vi "Scanner-XYZMove.vi"(5 "加速度":dbl=900.0, 7 "最高速":dbl=1000.0, 8 "Error In":errorcluster, 11 "X-Y-Z移動":dbl[](array[numeric])=[0.0, 0.0, 0.0]) -> (0 "Error Out":errorcluster, 1 "辨識結果(包含位置)":cluster{"讀取到時的位子":dbl, "辨識結果":string}[](array[cluster]), 2 "讀取到時的位子":dbl[](array[numeric]), 3 "辨識結果":string[](array[string]), 4 "辨識數量":i32, 6 "讀取機率":i32[](array[numeric]))   [LabVIEW 2019]
uses:
  <vilib>/Platform/TimedLoop/XDataNode/timing_clust.ctl
  <vilib>/Platform/TimedLoop/XDataNode/nitl_modes.ctl
  <vilib>/Platform/TimedLoop/XDataNode/wakeup.ctl
  9317ad16-1364-411d-9d7d-80c797a5b455.vi
  d1461482-5f26-4b15-89db-d86a902074c8.vi
  Variable/Lock-PID.vi
  Variable/Position.vi
  <vilib>/platform/TimedLoop/XDataNode/XDataNode.xnode
  <vilib>/Platform/TimedLoop/XDataNode/XDNodeRunTimeDep.lvlib
panel:
  out "讀取機率(折線圖)":i32[](graph)
  out "讀取機率":dbl[](array[slide]) scale=0.0..10.0
  out "三角形?":bool
  in  "Stop":bool
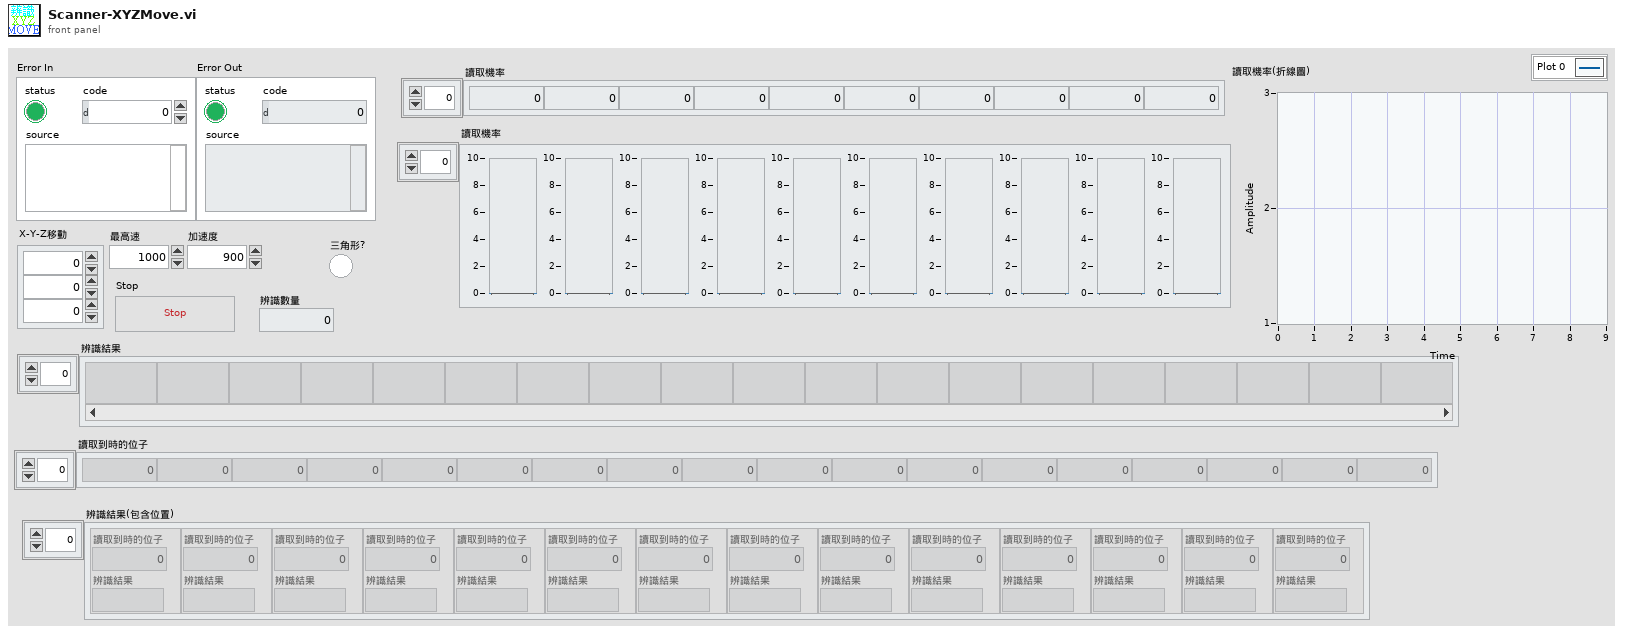
[diagram p1: front panel]
types:
  T1 = typedef "XDNodeRunTimeDep.lvlib/timing_clust.ctl" = cluster{"Expected End [f-1]":u64, "Actual End [f-1]":u64, "Finished Late? [f-1]":bool, "Expected End [i-1]":u64, "Actual End [i-1]":u64, "Finished Late? [i-1]":bool, "Expected Start [i]":u64, "Actual Start [i]":u64, "Expected Start [f]":u64, "Actual Start [f]":u64, "Source Name":string, "Structure Name":string, "Period":i64, "Deadline":i64, "Offset":i64, "Start":i64, "Priority":i32, "Timeout":i32, "Mode":T2, "Wakeup Reason":T3, "Error":errorcluster, "Source Type":string, "Secondary Source Type":string, "Global End Time":u64, "Global Start Time":u64, "Frame Duration":u64, "Iteration Duration":u64, "Assigned CPU":i32, "I/O Scan Engine Mode":u32}
  T2 = typedef "XDNodeRunTimeDep.lvlib/nitl_modes.ctl" = enum32{"No Change", "Process missed periods, maintain original phase", "Discard missed periods, maintain original phase", "Process missed periods, ignore original phase", "Discard missed periods, ignore original phase"}
  T3 = typedef "XDNodeRunTimeDep.lvlib/wakeup.ctl" = enum32{"Normal", "Aborted", "Asynchronous wakeup", "Timing source error", "Timed loop error", "Timeout"}
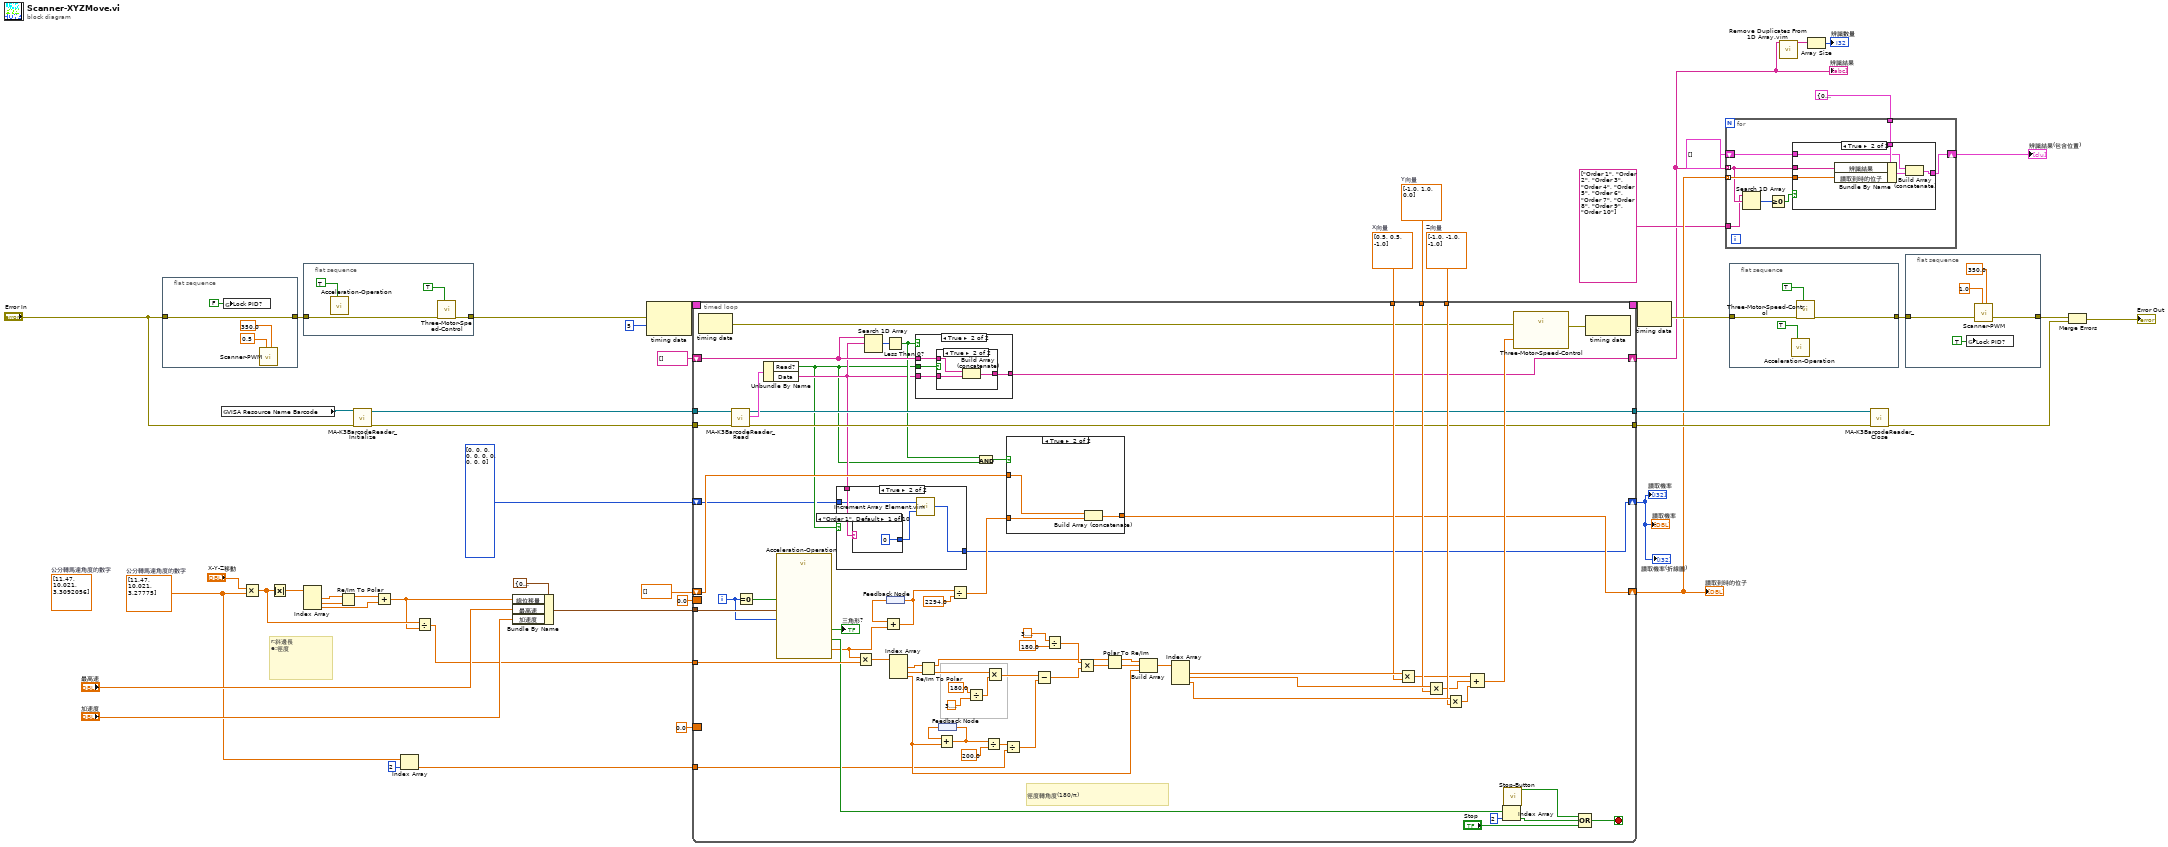
[diagram p0: block diagram]
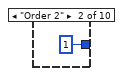
[diagram p4: hidden frame]
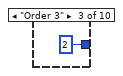
[diagram p5: hidden frame]
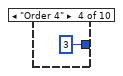
[diagram p6: hidden frame]
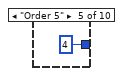
[diagram p7: hidden frame]
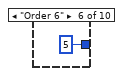
[diagram p8: hidden frame]
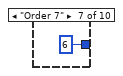
[diagram p9: hidden frame]
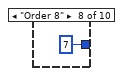
[diagram p10: hidden frame]
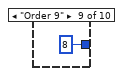
[diagram p11: hidden frame]
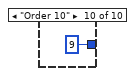
[diagram p12: hidden frame]
diagram:
  (unwired) dbl[] [11.47, 10.021, 3.3092056]  # 公分轉馬達角度的數字
  w29 = dbl[] [-1.0, -1.0, -1.0]  # Z向量
  w30 = dbl[] [-1.0, 1.0, 0.0]  # Y向量
  w31 = dbl[] [0.5, 0.5, -1.0]  # X向量
  w28 = dbl[] [11.47, 10.021, 3.27775]  # 公分轉馬達角度的數字
  # "r:斜邊長\ne:徑度"
  n1 = flat-sequence {
    tunnel: [w52] -> w24
    tunnel: "Error In" -> [w52]
    frame #0 {
      n2 = global write "Lock-PID.vi" "Lock PID?"(FALSE ("Lock PID?")) -> ()
      n3 = call "Scanner-PWM.vi"("Frequency [Hz]"=350.0, "Duty Cycle"=0.5) -> ()  [unwired: 9 in, 1 out]
    }
  }
  n4 = global read "Position.vi" "VISA Resource Name Barcode"() -> (w7:refnum<visa-resource-name>)
  n5 = Multiply(x="X-Y-Z移動", y=w28) -> (x*y=w35:dbl[])
  n6 = Absolute Value(x=w35) -> (abs(x)=w46:dbl[])
  n7 = Index Array(array=w46) -> (element #1=w42:dbl, element #2=w47:dbl, element #3=w43:dbl)  [unwired: 3 in]
  n8 = flat-sequence {
    tunnel: w24 -> [w56]
    tunnel: [w55] -> w34
    frame #0 {
      n9 = call "Acceleration-Operation.vi"("Reset"=TRUE) -> ()  [unwired: 8 in, 3 out]
      n10 = call "Three-Motor-Speed-Control.vi"("Reset"=TRUE, "Error In"=w56) -> ("Error Out"=w55:errorcluster)  [unwired: 9 in]
    }
  }
  n11 = Re/Im To Polar(2:w47, 3:w42) -> (1:w44:dbl)  [unwired: 1 out]
  n12 = call "MA-K3BarcodeReader_Initialize.vi"("Error In"="Error In", "掃碼機串口"=w7) -> ("Error Out"=w15:errorcluster, "VISA Resource"=w14:refnum<visa-resource-name>)  [unwired: 8 in]
  n13 = Add(x=w44, y=w43) -> (x+y=w23:dbl)
  n14 = Index Array(array=w28, index=2) -> (element=w27:dbl)
  n15 = Divide(x=w35, y=w23) -> (x/y=w36:dbl[])
  n16 = Bundle By Name(cluster=cluster{"總位移量":dbl, "最高速":dbl, "加速度":dbl} {"總位移量"=0.0, "最高速"=0.0, "加速度"=0.0} ("計算設置"), "總位移量"=w23, "最高速"="最高速", "加速度"="加速度") -> (w37:cluster{"總位移量":dbl, "最高速":dbl, "加速度":dbl})
  n17 = node-c288(w34, i64 5 ("Period")) -> (w49:T1)
  n18 = timed-loop "Timed Loop" {
    timing: w49 -> [_]
    timing-out: [_] -> w48
    tunnel: w37 -> [w125]
    tunnel: w36 -> [w124]
    border: 0.0 -> [_]
    tunnel: w31 -> [w94]
    tunnel: w30 -> [w92]
    tunnel: w29 -> [w90]
    tunnel: w27 -> [w82]
    border: 0.0 -> [_]
    shift-right: [w73] -> w12
    shift-left: dbl[] [] -> [w72]
    tunnel: [w69] -> w18
    tunnel: [w68] -> w17
    shift-right: [w70] -> w5
    shift-left: string[] [] -> [w65]
    tunnel: w15 -> [w67]
    tunnel: w14 -> [w66]
    shift-right: [w58] -> w1
    shift-left: i32[] [0, 0, 0, 0, 0, 0, 0, 0, 0, 0] -> [w59]
    i -> [w122]
    stop <- w120 stop-if-true
    # "徑度轉角度(180/π)"
    n19 = node-c288() -> (w85:errorcluster)  [unwired: 1 in]
    n20 = call "MA-K3BarcodeReader_Read.vi"("error in (no error)"=w67, "VISA Reference"=w66) -> ("error out"=w69:errorcluster, "Result"=w71:cluster{"Read?":bool, "Data":string}, "VISA Reference"=w68:refnum<visa-resource-name>)  [unwired: 7 in]
    n21 = Equal To 0?(x=w122) -> (x = 0?=w123:bool)
    n22 = Unbundle By Name(w71) -> ("Read?"=w60:bool, "Data"=w61:string)
    n23 = call "Acceleration-Operation.vi"("Reset"=w123, "迴圈( I )"=w122, "計算設置"=w125) -> ("完成?"=w119:bool[], "速度"=w78:dbl, "三角形?"=→"三角形?":bool)  [unwired: 6 in]
    n24 = case shown="True" w60 {
      tunnel: w61 -> [_ w130]
      tunnel: w59 -> [w126 w129]
      tunnel: [w126 w127] -> w58
      frame False {
      }
      frame True {
        n25 = case shown="\"Order 1\", Default" w130 {
          tunnel: [0 1 2 3 4 5 6 7 8 9] -> w128
          frame "Order 1", Default {
          }
          frame "Order 2" {
          }
          frame "Order 3" {
          }
          frame "Order 4" {
          }
          frame "Order 5" {
          }
          frame "Order 6" {
          }
          frame "Order 7" {
          }
          frame "Order 8" {
          }
          frame "Order 9" {
          }
          frame "Order 10" {
          }
        }
        n26 = call "Increment Array Element.vim"("index"=w128, "array in"=w129) -> ("array out"=w127:i32[])
      }
    }
    n27 = Multiply(x=w78, y=w124) -> (x*y=w116:dbl[])
    n28 = Search 1D Array(1D array=w65, element=w61) -> (index of element=w64:i32)  [unwired: 1 in]
    n29 = Less Than 0?(x=w64) -> (x < 0?=w62:bool)
    n30 = feedback #1() -> (w77:dbl)
    n31 = Add(x=w77, y=w78) -> (x+y=w76:dbl)
    n32 = feedback-in #1(w76) -> ()
    n33 = Index Array(array=w116) -> (element #1=w115:dbl, element #2=w114:dbl, element #3=w97:dbl)  [unwired: 3 in]
    n34 = case shown="True" w62 {
      tunnel: w61 -> [_ w145]
      tunnel: w60 -> [_ w144]
      tunnel: [w141 w143] -> w70
      tunnel: w65 -> [w141 w142]
      frame False {
      }
      frame True {
        n35 = case shown="True" w144 {
          tunnel: w145 -> [_ w149]
          tunnel: [w146 w148] -> w143
          tunnel: w142 -> [w146 w147]
          frame False {
          }
          frame True {
            n36 = Build Array (concatenate)(w147, w149) -> (w148:string[])
          }
        }
      }
    }
    n37 = Re/Im To Polar(2:w114, 3:w115) -> (0:w113:dbl, 1:w100:dbl)
    n38 = feedback #2() -> (w109:dbl)
    n39 = Add(x=w109, y=w97) -> (x+y=w108:dbl)
    n40 = feedback-in #2(w108) -> ()
    n41 = Divide(x=w76, y=2294.0) -> (x/y=w74:dbl)
    n42 = Divide(x=180.0, y=3.141592653589793) -> (x/y=w110:dbl)
    n43 = And(x=w62, y=w60) -> (x .and. y?=w63:bool)
    n44 = Divide(x=w108, y=200.0) -> (x/y=w84:dbl)
    n45 = Multiply(x=w113, y=w110) -> (x*y=w106:dbl)
    n46 = Divide(x=w84, y=w82) -> (x/y=w83:dbl)
    n47 = case shown="True" w63 {
      tunnel: w74 -> [_ w153]
      tunnel: [w150 w152] -> w73
      tunnel: w72 -> [w150 w151]
      frame False {
      }
      frame True {
        n48 = Build Array (concatenate)(w151, w153) -> (w152:dbl[])
      }
    }
    n49 = Subtract(x=w106, y=w83) -> (x-y=w102:dbl)
    n50 = Divide(x=3.141592653589793, y=180.0 ("x")) -> (x/y=w103:dbl)
    n51 = Multiply(x=w103, y=w102) -> (x*y=w101:dbl)
    n52 = Polar To Re/Im(2:w101, 3:w100) -> (0:w98:dbl, 1:w99:dbl)
    n53 = Build Array(w99, w98, w97) -> (w96:dbl[])
    n54 = Index Array(array=w96) -> (element #1=w95:dbl, element #2=w93:dbl, element #3=w91:dbl)  [unwired: 3 in]
    n55 = Multiply(x=w95, y=w94) -> (x*y=w89:dbl[])
    n56 = Multiply(x=w93, y=w92) -> (x*y=w88:dbl[])
    n57 = Multiply(x=w91, y=w90) -> (x*y=w87:dbl[])
    n58 = Compound Arithmetic op=ADD(w89, w88, w87) -> (w79:dbl[])
    n59 = Index Array(array=w119, index=2) -> (element=w80:bool)
    n60 = call "Stop-Button.vi"() -> ("顯示按下?"=w81:bool)  [unwired: 10 in, 1 out]
    n61 = call "Three-Motor-Speed-Control.vi"("Error In"=w85, "速度(秒/度)"=w79) -> ("Error Out"=w86:errorcluster)  [unwired: 9 in]
    n62 = Compound Arithmetic op=OR(w81, w80, "Stop") -> (w120:bool)
    n63 = node-c288(w86) -> ()  [unwired: 1 out]
  }
  "辨識結果" <- w5
  "讀取到時的位子" <- w12
  "讀取機率" <- w1
  "讀取機率" <- w1
  "讀取機率(折線圖)" <- w1
  n64 = node-c288(w48) -> (w33:errorcluster)
  n65 = for {
    tunnel: w5 -> [w162] mode=indexing
    tunnel: cluster{"讀取到時的位子":dbl, "辨識結果":string} {"讀取到時的位子"=0.0, "辨識結果"=""} ("input cluster") -> [w166]
    tunnel: w12 -> [w165] mode=indexing
    shift-right: [w164] -> w9
    shift-left: cluster{"讀取到時的位子":dbl, "辨識結果":string}[] [] -> [w163]
    tunnel: string[] ["Order 1", "Order 2", "Order 3", "Order 4", "Order 5", "Order 6", "Order 7", "Order 8", "Order 9", "Order 10"] -> [w161]
    n66 = Search 1D Array(1D array=w161, element=w162) -> (index of element=w159:i32)  [unwired: 1 in]
    n67 = Greater Or Equal To 0?(x=w159) -> (x >= 0?=w160:bool)
    n68 = case shown="True" w160 {
      tunnel: w162 -> [_ w173]
      tunnel: w166 -> [_ w172]
      tunnel: w165 -> [_ w171]
      tunnel: [w167 w169] -> w164
      tunnel: w163 -> [w167 w168]
      frame False {
      }
      frame True {
        n69 = Bundle By Name(cluster=w172, "辨識結果"=w173, "讀取到時的位子"=w171) -> (w170:cluster{"讀取到時的位子":dbl, "辨識結果":string})
        n70 = Build Array (concatenate)(w168, w170) -> (w169:cluster{"讀取到時的位子":dbl, "辨識結果":string}[])
      }
    }
  }
  "辨識結果(包含位置)" <- w9
  n71 = flat-sequence {
    tunnel: w33 -> [w176]
    tunnel: [w175] -> w25
    frame #0 {
      n72 = call "Acceleration-Operation.vi"("Reset"=TRUE) -> ()  [unwired: 8 in, 3 out]
      n73 = call "Three-Motor-Speed-Control.vi"("Reset"=TRUE, "Error In"=w176) -> ("Error Out"=w175:errorcluster)  [unwired: 9 in]
    }
  }
  n74 = call "Remove Duplicates From 1D Array.vim"("array"=w5) -> ("array with duplicates removed"=w4:string[])  [unwired: 10 in]
  n75 = Array Size(array=w4) -> (size(s)=→"辨識數量":i32)
  n76 = call "MA-K3BarcodeReader_Close.vi"("Error In"=w18, "VISA Resource"=w17) -> ("Error Out"=w11:errorcluster)  [unwired: 9 in]
  n77 = flat-sequence {
    tunnel: [w180] -> w22
    tunnel: w25 -> [w180]
    frame #0 {
      n78 = global write "Lock-PID.vi" "Lock PID?"(TRUE ("Lock PID?")) -> ()
      n79 = call "Scanner-PWM.vi"("Frequency [Hz]"=350.0, "Duty Cycle"=1.0) -> ()  [unwired: 9 in, 1 out]
    }
  }
  n80 = Merge Errors(w22, w11) -> (→"Error Out":errorcluster)
